vi "Untitled 2.vi"() -> ()   [LabVIEW 2019]
uses:
  <userlib>/LevyLab/Instrument Framework/Instrument Types/Lockin/Instrument.LockinAPI.lvclass
  C:/Program Files (x86)/National Instruments/LabVIEW 2019/user.lib/LevyLab/Instrument Framework/Instrument/Instrument.lvclass
  <userlib>/LevyLab/Krohn Hite 7008/Inst.Krohn-Hite-7008/Inst.Krohn-Hite-7008.lvclass
  <userlib>/LevyLab/Lockin-Multichannel/Instrument.Lockin/Instrument.Lockin.lvclass
  <userlib>/LevyLab/Instrument Framework/Instrument/Instrument.lvclass
  C:/Program Files (x86)/National Instruments/LabVIEW 2019/user.lib/LevyLab/Instrument Framework/Instrument Types/Lockin/Instrument.LockinAPI.lvclass
  C:/Program Files (x86)/National Instruments/LabVIEW 2019/vi.lib/JKI/JKI SMO/SMO/SMO.lvclass
panel:
  out "ACK":string
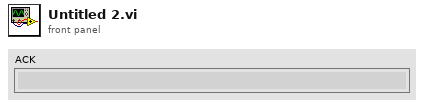
[diagram p1: front panel]
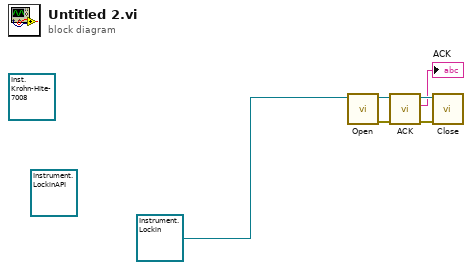
[diagram p0: block diagram]
diagram:
  (unwired) refnum<class "Instrument.LockinAPI.lvclass"> refnum ("Instrument.LockinAPI in")
  (unwired) refnum<class "Inst.Krohn-Hite-7008.lvclass"> refnum ("Inst.Krohn-Hite-7008 in")
  n1 = call-dynamic "Open.vi"("Instrument.Lockin in"=refnum<class "Instrument.Lockin.lvclass"> refnum) -> ("error out"=w5:errorcluster, "Instrument.Lockin out"=w6:refnum<class "Instrument.Lockin.lvclass">)  [unwired: 9 in]
  n2 = call <userlib>:"ACK.vi"("error in (no error)"=w5, "Instrument in"=w6) -> ("error out"=w3:errorcluster, "ACK"=→"ACK":string, "Instrument in"=w4:refnum<class "Instrument.Lockin.lvclass">)  [unwired: 7 in]
  n3 = call-dynamic "Close.vi"("error in (no error)"=w3, "Instrument.Lockin in"=w4) -> ()  [unwired: 8 in, 2 out]
